vi "Write Buffer Size.vi"(8 "error in (no error)":errorcluster, 10 "Buffer Size":i32=4096, 11 "Network Stream in":refnum<class "Network Stream.lvclass">) -> (0 "error out":errorcluster, 3 "Network Stream out":refnum<class "Network Stream.lvclass">)   [LabVIEW 2014, in "Network Stream.lvlib" / "Network Stream.lvclass"]
uses:
  Network Stream.lvclass
  Network Stream.lvclass/Network Stream.ctl
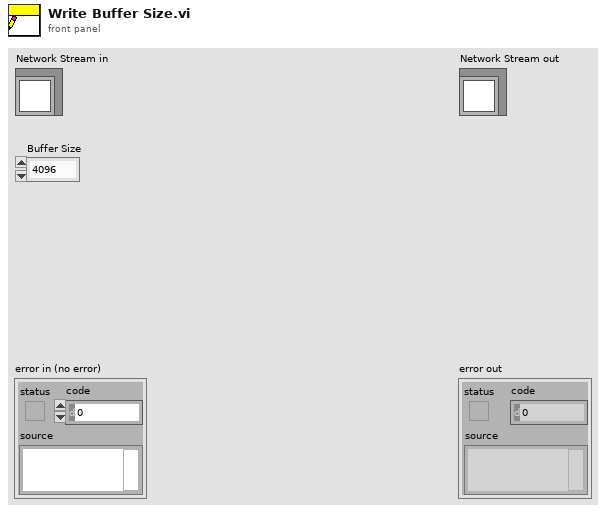
[diagram p1: front panel]
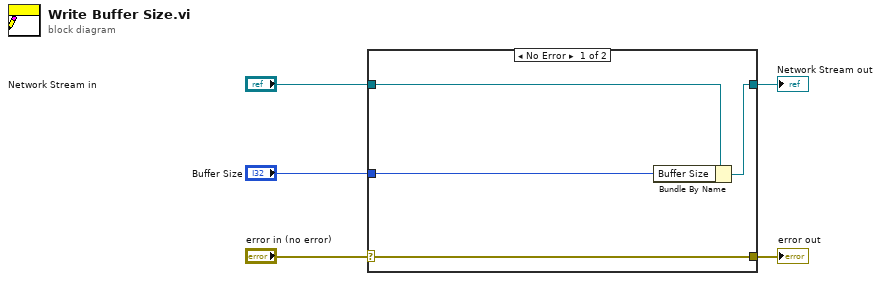
[diagram p0: block diagram]
diagram:
  n1 = case shown="No Error" "error in (no error)" {
    selector: "error in (no error)" -> [w9 w10]
    tunnel: [w9 w10] -> w4
    tunnel: [w7 w11] -> w2
    tunnel: "Network Stream in" -> [w8 w11]
    tunnel: "Buffer Size" -> [w6 _]
    frame No Error {
      n2 = Bundle By Name(cluster=w8, "Buffer Size"=w6) -> (w7:refnum<class "Network Stream.lvclass">)
    }
    frame Error {
    }
  }
  "error out" <- w4
  "Network Stream out" <- w2
